vi "roaming VI.vi"(0 "scan angle":sgl=90.0, 5 "step angle":sgl=4.0, 12 "stop":bool) -> (2 "sensor data":cluster{dbl[], dbl[]}(graph)={[-0.048166929668633715], [0.4724490056471417]}, 3 "Array":u32[][](array[colorbox]), 4 "sensor":bool, 6 "left motor":bool, 8 "right motor":bool, 10 "x":dbl, 13 "map reference out":refnum<data-value>, 14 "velocity":dbl, 15 "y":dbl)   [LabVIEW 2011]
uses:
  <vilib>/robotics/Navigation/shared/WorldMap/OccupancyGridWorldMap/NI_Robotics_OccupancyGridWorldMap.lvclass
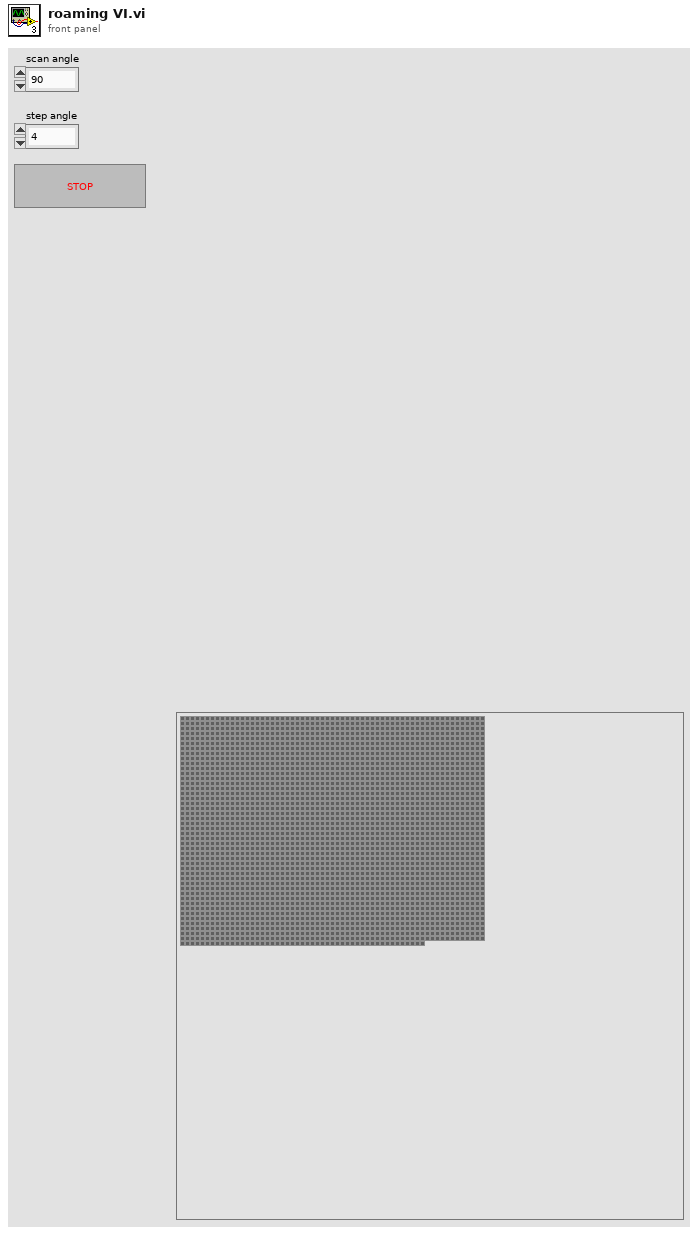
[diagram p1: front panel]
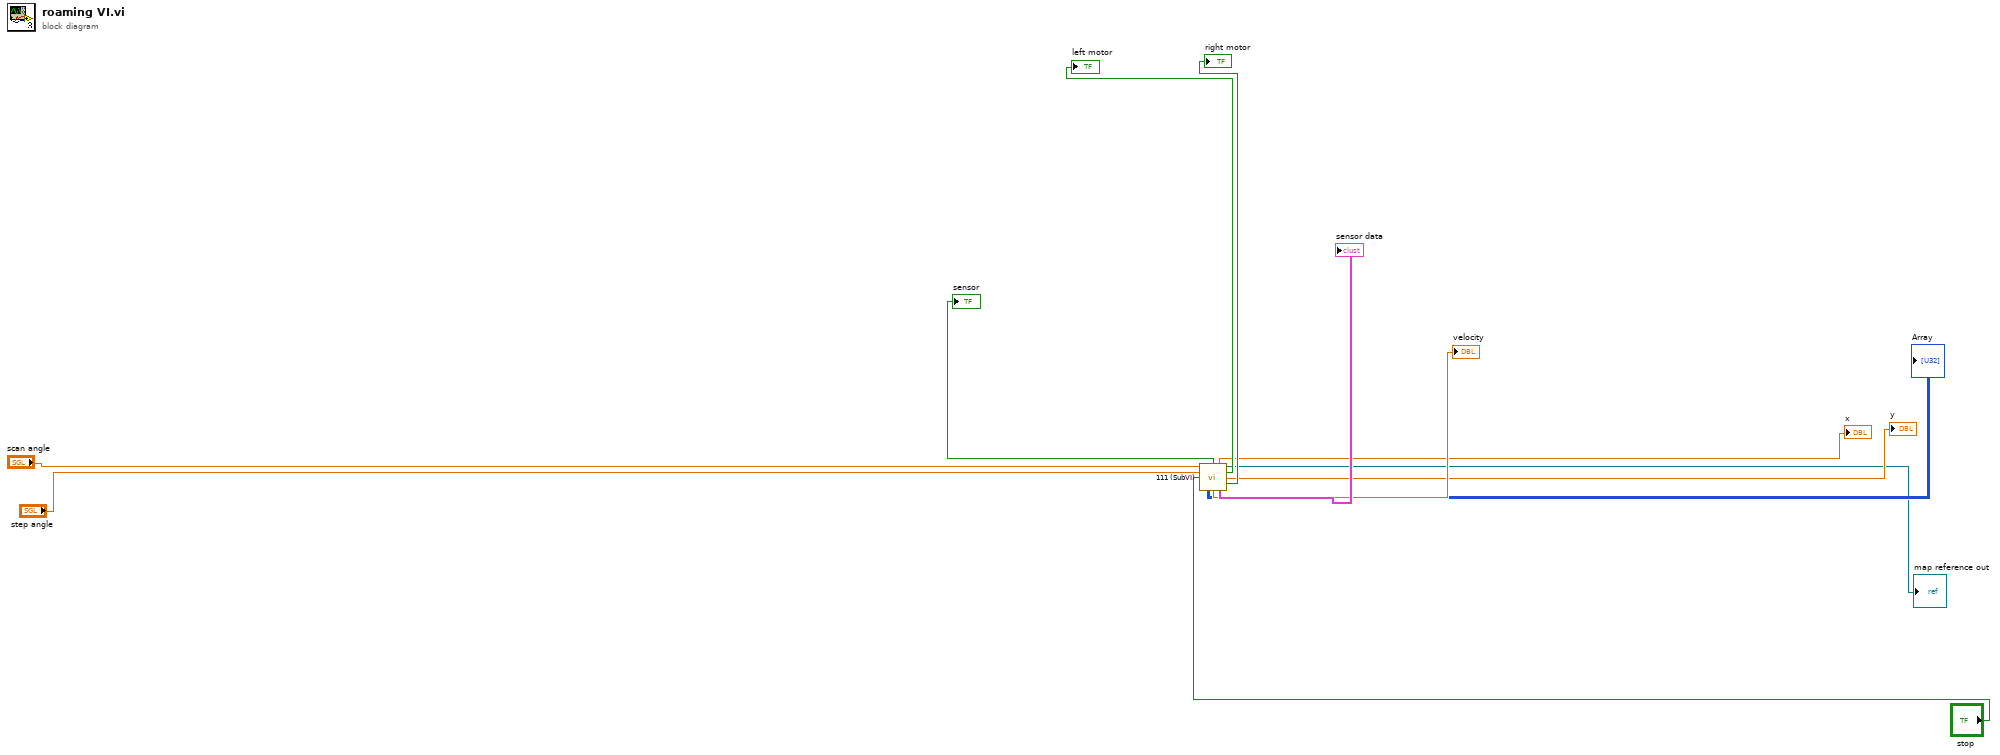
[diagram p0: block diagram]
diagram:
  n1 = call "111 (SubVI).vi"("scan angle"="scan angle", "step angle"="step angle", "stop"="stop") -> ("sensor"=→"sensor":bool, "x"=→"x":dbl, "Data Value Reference out"=→"map reference out":refnum<data-value>, "left motor"=→"left motor":bool, "y"=→"y":dbl, "right motor"=→"right motor":bool, "Array"=→"Array":u32[][], "velocity"=→"velocity":dbl, "sensor data"=→"sensor data":cluster{dbl[], dbl[]})  [unwired: 4 in]
